vi "Initialise Motion At Random Position With Angle.vi"(4 "Initial Velocity [m/s]":sgl=1.0 format="%#_13g", 5 "Field Size":T1={"x"=500.0, "y"=500.0}, 8 "Maximum Velocity [m/s]":sgl=inf, 9 "Acceleration [m/s/s]":sgl=10.0 format="%.3g", 10 "Turn Rate [deg/s]":sgl=90.0 format="%.3g", 11 "Element in":refnum<class "Element.lvclass">) -> (3 "Element out":refnum<class "Element.lvclass">)   [LabVIEW 2021, in "Element.lvclass"]
uses:
  Element.lvclass
  Element.lvclass/Element.ctl
  Motion/Motion.lvclass
  Math/Vec2.ctl
  Math/Math.lvlib
  <vilib>/numeric/Random Number (Range) DBL.vi
panel:
  in  "Initial Heading [deg]":sgl=1.0 format="%#_13g"
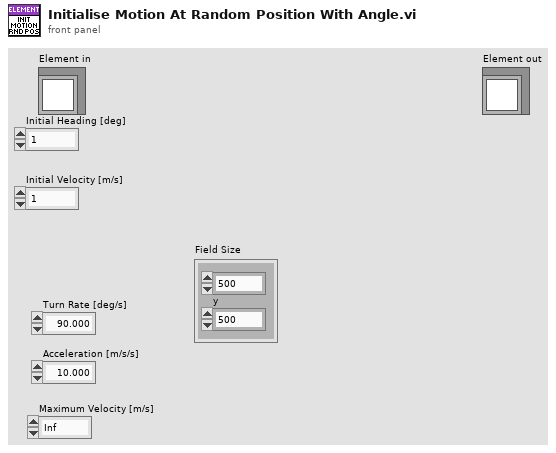
[diagram p1: front panel]
types:
  T1 = typedef "Math.lvlib/Vec2.ctl" = cluster{"x":sgl, "y":sgl}
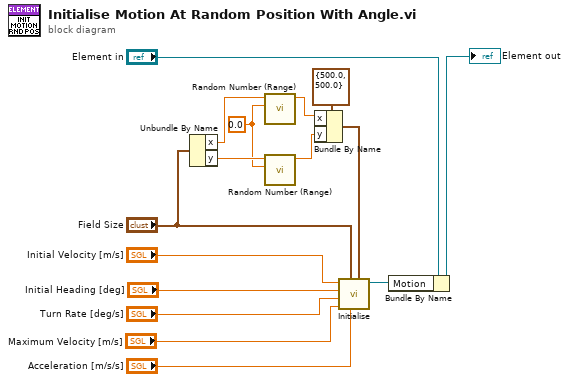
[diagram p0: block diagram]
diagram:
  w3 = 0.0 ("Low")
  n1 = Unbundle By Name("Field Size") -> ("x"=w5:sgl, "y"=w4:sgl)
  n2 = call-poly <vilib>:"Random Number (Range).vi"("lower bound (0)"=w3, "upper bound (100)"=w5) -> ("number"=w7:dbl)  [unwired: 9 in]
  n3 = call-poly <vilib>:"Random Number (Range).vi"("lower bound (0)"=w3, "upper bound (100)"=w4) -> ("number"=w6:dbl)  [unwired: 9 in]
  n4 = Bundle By Name(cluster=T1 {"x"=500.0, "y"=500.0} ("Field Size"), "x"=w7, "y"=w6) -> (w8:T1)
  n5 = call "Initialise.vi"("Initial Position"=w8, "Acceleration [m/s/s]"="Acceleration [m/s/s]", "Field Size"="Field Size", "Maximum Velocity [m/s]"="Maximum Velocity [m/s]", "Turn Rate [deg/s]"="Turn Rate [deg/s]", "Initial Heading [deg]"="Initial Heading [deg]", "Initial Velocity [m/s]"="Initial Velocity [m/s]") -> ("Motion out"=w15:refnum<class "Motion.lvclass">)  [unwired: 4 in]
  n6 = Bundle By Name(cluster="Element in", "Motion"=w15) -> (→"Element out":refnum<class "Element.lvclass">)
